vi "Create_AO_Z_WF.vi"(8 "error in":errorcluster) -> (0 "error out":errorcluster)   [LabVIEW 2025]
uses:
  <vilib>/Waveform/WDTOps.llb/WDT Append Waveforms DBL.vi
panel:
  out "Illumination analog waveforms":waveform(dbl)(graph) caption="Output Waveform"
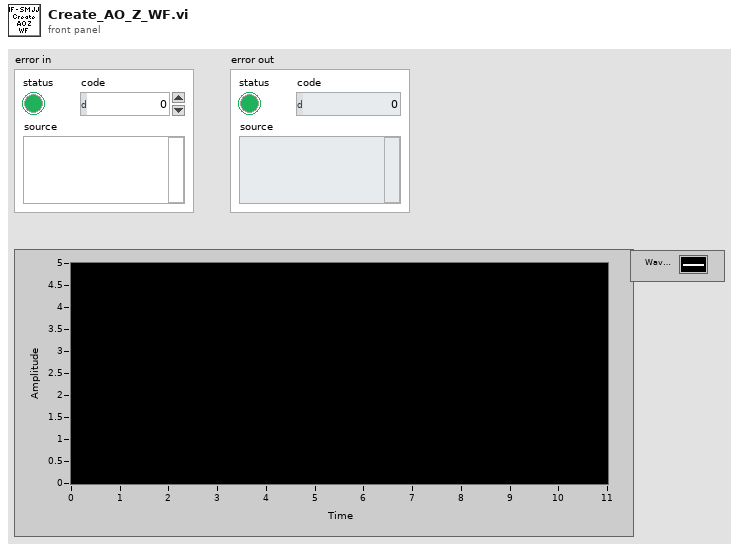
[diagram p1: front panel]
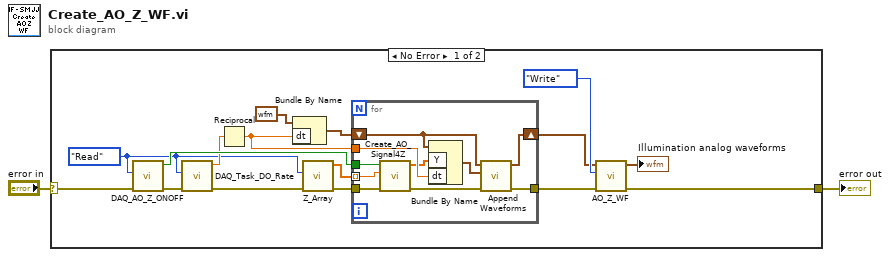
[diagram p0: block diagram]
diagram:
  n1 = case shown="No Error" "error in" {
    selector: "error in" -> [w18 w29]
    tunnel: [w17 w29] -> w1
    frame No Error {
      w4 = enum16{"Write", "Read"}."Read" ("Action")
      n2 = call "DAQ_AO_Z_ONOFF.vi"("error in"=w18, "Action"=w4) -> ("error out"=w14:errorcluster, "ON / OFF"=w15:bool)  [unwired: 8 in]
      n3 = call "DAQ_Task_DO_Rate.vi"("error in"=w14, "Action"=w4) -> ("error out"=w3:errorcluster, "DO_Rate"=w13:dbl)  [unwired: 8 in]
      n4 = Reciprocal(x=w13) -> (1/x=w8:dbl)
      n5 = Bundle By Name(cluster=waveform(dbl) {"t0"=timestamp(0 s since 1904-01-01), "dt"=0.001, "Y"=[]} ("waveform out"), "dt"=w8) -> (w7:waveform(dbl))
      n6 = call "Z_Array.vi"("error in"=w3, "Action"=w4) -> ("error out"=w11:errorcluster, "Z_Array"=w12:dbl[])  [unwired: 8 in]
      n7 = for {
        tunnel: [w21] -> w5
        tunnel: w15 -> [w28]
        tunnel: w8 -> [w27]
        tunnel: w12 -> [w25] mode=indexing
        tunnel: w11 -> [w24]
        shift-right: [w22] -> w6
        shift-left: w7 -> [w19]
        n8 = call "Create_AO_Signal4Z.vi"("error in"=w24, "AO Amplitude"=w25, "ON / OFF"=w28) -> ("error out"=w23:errorcluster, "WF"=w26:dbl[])  [unwired: 7 in]
        n9 = Bundle By Name(cluster=w19, "Y"=w26, "dt"=w27) -> (w20:waveform(dbl))
        n10 = call-poly <vilib>:"Append Waveforms.vi"("error in (no error)"=w23, "waveform B"=w20, "waveform A"=w19) -> ("error out"=w21:errorcluster, "waveform out"=w22:waveform(dbl))  [unwired: 7 in]
      }
      n11 = call "AO_Z_WF.vi"("error in"=w5, "Action"=enum16{"Write", "Read"}."Write", "AO Z WF"=w6) -> ("error out"=w17:errorcluster, "AO Z WF"=→"Illumination analog waveforms":waveform(dbl))  [unwired: 7 in]
    }
    frame Error {
    }
  }
  "error out" <- w1
